vi "Get configuration chain.vi"(8 "error in (no error)":errorcluster, 11 "ImageStackBase in":refnum<class "ImageStack.lvclass">) -> (0 "error out":errorcluster, 1 "class name":string[](array[string]), 2 "configuration chain":variant[](array[variant]), 3 "ImageStackBase out":refnum<class "ImageStack.lvclass">)   [LabVIEW 2012, in "ImageStack.lvclass"]
doc: "Returns an array of variants containing the configuration clusters of each class in the inheritance chain (lowest child class first), together with an array of all class names in the inheritance chain.\n\nFor classes without configuration cluster, the configuration chain contains empty variants."
uses:
  ImageStack.lvclass
  <vilib>/Distrio/Murmex/Murmex/Murmex.lvclass
  ImageStack.lvclass/ImageStack.ctl
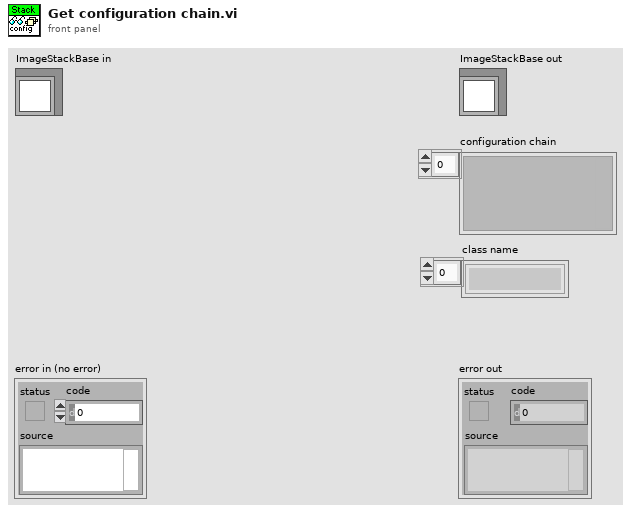
[diagram p1: front panel]
types:
  T1 = typedef "ImageStack.lvclass/configuration_cluster.ctl" = cluster{"Camera component name":string, "Stages component name":string, "AOTF component name":string}
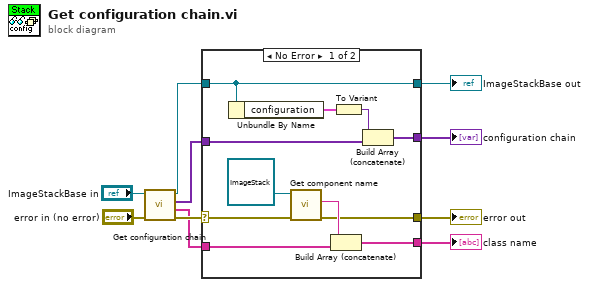
[diagram p0: block diagram]
diagram:
  n1 = call-parent "Get configuration chain.vi"("error in (no error)"="error in (no error)", "MurmexBase in"="ImageStackBase in") -> ("error out"=w8:errorcluster, "class name"=w7:string[], "configuration chain"=w3:variant[], "MurmexBase out"=w5:refnum<class "ImageStack.lvclass">)  [unwired: 6 in]
  n2 = case shown="No Error" w8 {
    selector: w8 -> [w21 w23]
    tunnel: w7 -> [w18 w22]
    tunnel: [w17 w22] -> w6
    tunnel: [w16 w25] -> w4
    tunnel: w5 -> [w16 w25]
    tunnel: w3 -> [w13 w24]
    tunnel: [w12 w24] -> w2
    tunnel: [w11 w23] -> w1
    frame No Error {
      n3 = Unbundle By Name(w16) -> ("configuration"=w15:T1)
      n4 = call <vilib>:"Get component name.vi"("error in (no error)"=w21, "Murmex in"=refnum<class "ImageStack.lvclass"> refnum ("ImageStack")) -> ("error out"=w11:errorcluster, "component name"=w19:string)  [unwired: 7 in, 1 out]
      n5 = Build Array (concatenate)(w19, w18) -> (w17:string[])
      n6 = To Variant(anything=w15) -> (Variant=w14:variant)
      n7 = Build Array (concatenate)(w14, w13) -> (w12:variant[])
    }
    frame Error {
    }
  }
  "error out" <- w1
  "ImageStackBase out" <- w4
  "configuration chain" <- w2
  "class name" <- w6
